vi "waveform_conversion_v2.vi"(6 "sample length":i32, 9 "y":dbl, 10 "y 2":dbl, 11 "data":waveform(dbl)[](array[waveform])) -> (3 "mean":dbl)   [LabVIEW 2026]
uses:
  <vilib>/ptbypt/NI_PtbyPt.lvlib
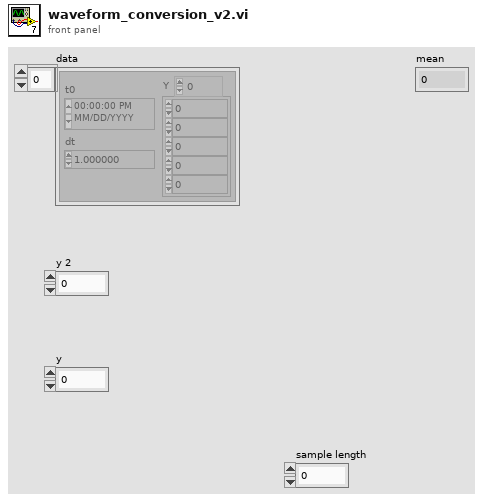
[diagram p1: front panel]
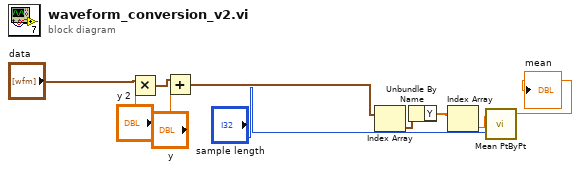
[diagram p0: block diagram]
diagram:
  n1 = Multiply(x="data", y="y 2") -> (x*y=w4:waveform(dbl)[])
  n2 = Add(x=w4, y="y") -> (x+y=w10:waveform(dbl)[])
  n3 = Index Array(array=w10) -> (element=w7:waveform(dbl))  [unwired: 1 in]
  n4 = Unbundle By Name(w7) -> ("Y"=w8:dbl[])
  n5 = Index Array(array=w8) -> (element=w9:dbl)  [unwired: 1 in]
  n6 = call <vilib>:"Mean PtByPt.vi"("x"=w9, "sample length"="sample length") -> ("mean"=→"mean":dbl)  [unwired: 2 in, 1 out]
